vi "PD500 - PWM test cleanup_v2.vi"(0 "Control Board VISA":refnum<visa-resource-name>="ControlBoard", 1 "HMP VISA":refnum<visa-resource-name>, 2 "Board Selector":T1, 5 "error in (no error) 2":errorcluster) -> (12 "T6":dbl[](array[numeric]), 13 "T5":dbl[](array[numeric]), 15 "T4":dbl[](array[numeric]), 16 "T3":dbl[](array[numeric]), 17 "T2":dbl[](array[numeric]), 18 "T1":dbl[](array[numeric]), 19 "error out":errorcluster)   [LabVIEW 2022 SP3]
uses:
  Serial Board Com/Board Select.ctl
  HMP4000 Communication/HMP4040_ChannelControlAutomatic.ctl
  <vilib>/DAQmx/read.llb/DAQmx Read (Analog 1D Wfm NChan NSamp).vi
  <vilib>/DAQmx/miscellaneous.llb/DAQmx Fill In Error Info.vi
panel:
  out "subarray 12":dbl[](array[numeric])
  out "subarray 11":dbl[](array[numeric])
  out "subarray 10":dbl[](array[numeric])
  out "subarray 9":dbl[](array[numeric])
  out "subarray 8":dbl[](array[numeric])
  out "subarray 7":dbl[](array[numeric])
  out "subarray 6":dbl[](array[numeric])
  out "subarray 5":dbl[](array[numeric])
  out "subarray 4":dbl[](array[numeric])
  out "subarray 3":dbl[](array[numeric])
  out "subarray 2":dbl[](array[numeric])
  out "subarray":dbl[](array[numeric])
  out "Duty Cycle VISA Write":string[](array[string])
  out "Analysis Leg":i32
  out "Waveforms":T2
  out "Active Leg":i32
  # "Hugo: Needs Further Cleanup Regarding Data"
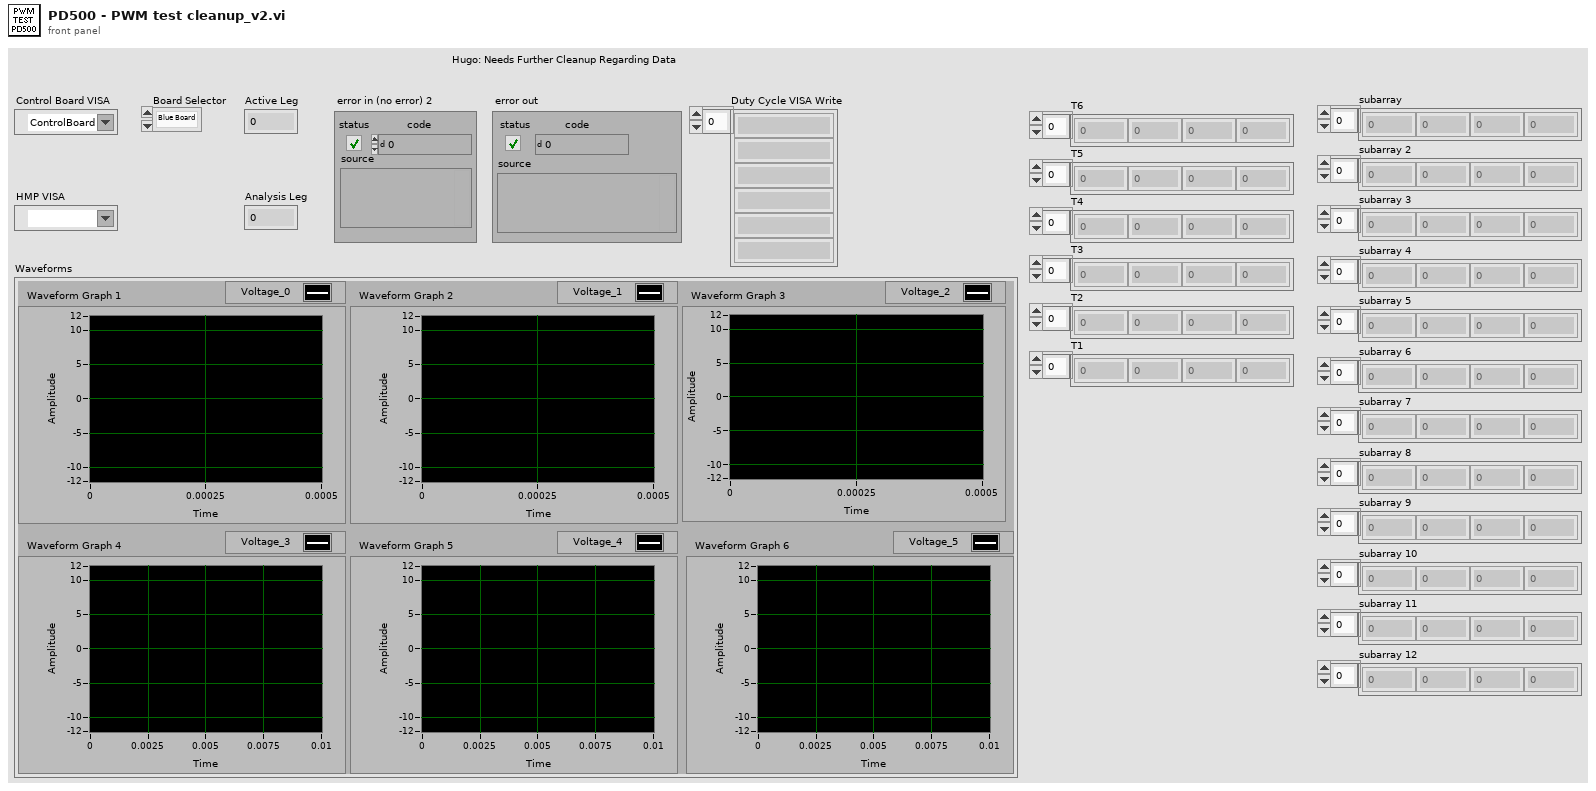
[diagram p1: front panel]
types:
  T1 = typedef "Board Select.ctl" = enum16{"Blue Board", "Green Board"}
  T2 = cluster{"Waveform Graph 1":waveform(dbl), "Waveform Graph 2":waveform(dbl), "Waveform Graph 3":waveform(dbl), "Waveform Graph 4":waveform(dbl), "Waveform Graph 5":waveform(dbl), "Waveform Graph 6":waveform(dbl)}
  T3 = typedef "HMP4040_ChannelControlAutomatic.ctl" = enum16{"Off", "Control Power", "HMP2020 Control + DC32V", "HMP2020 Control + DC8V", "HMP4040 Control + DC32V", "HMP4040 Control +DC8V", "HMP4040 Ch2 24V 4A"}
  T4 = cluster{"data[0]":waveform(dbl), "data[1]":waveform(dbl), "data[2]":waveform(dbl), "data[3]":waveform(dbl), "data[4]":waveform(dbl), "data[5]":waveform(dbl)}
  T5 = typedef "NI_Matrix.lvlib/RealMatrix.ctl" = dbl[][]
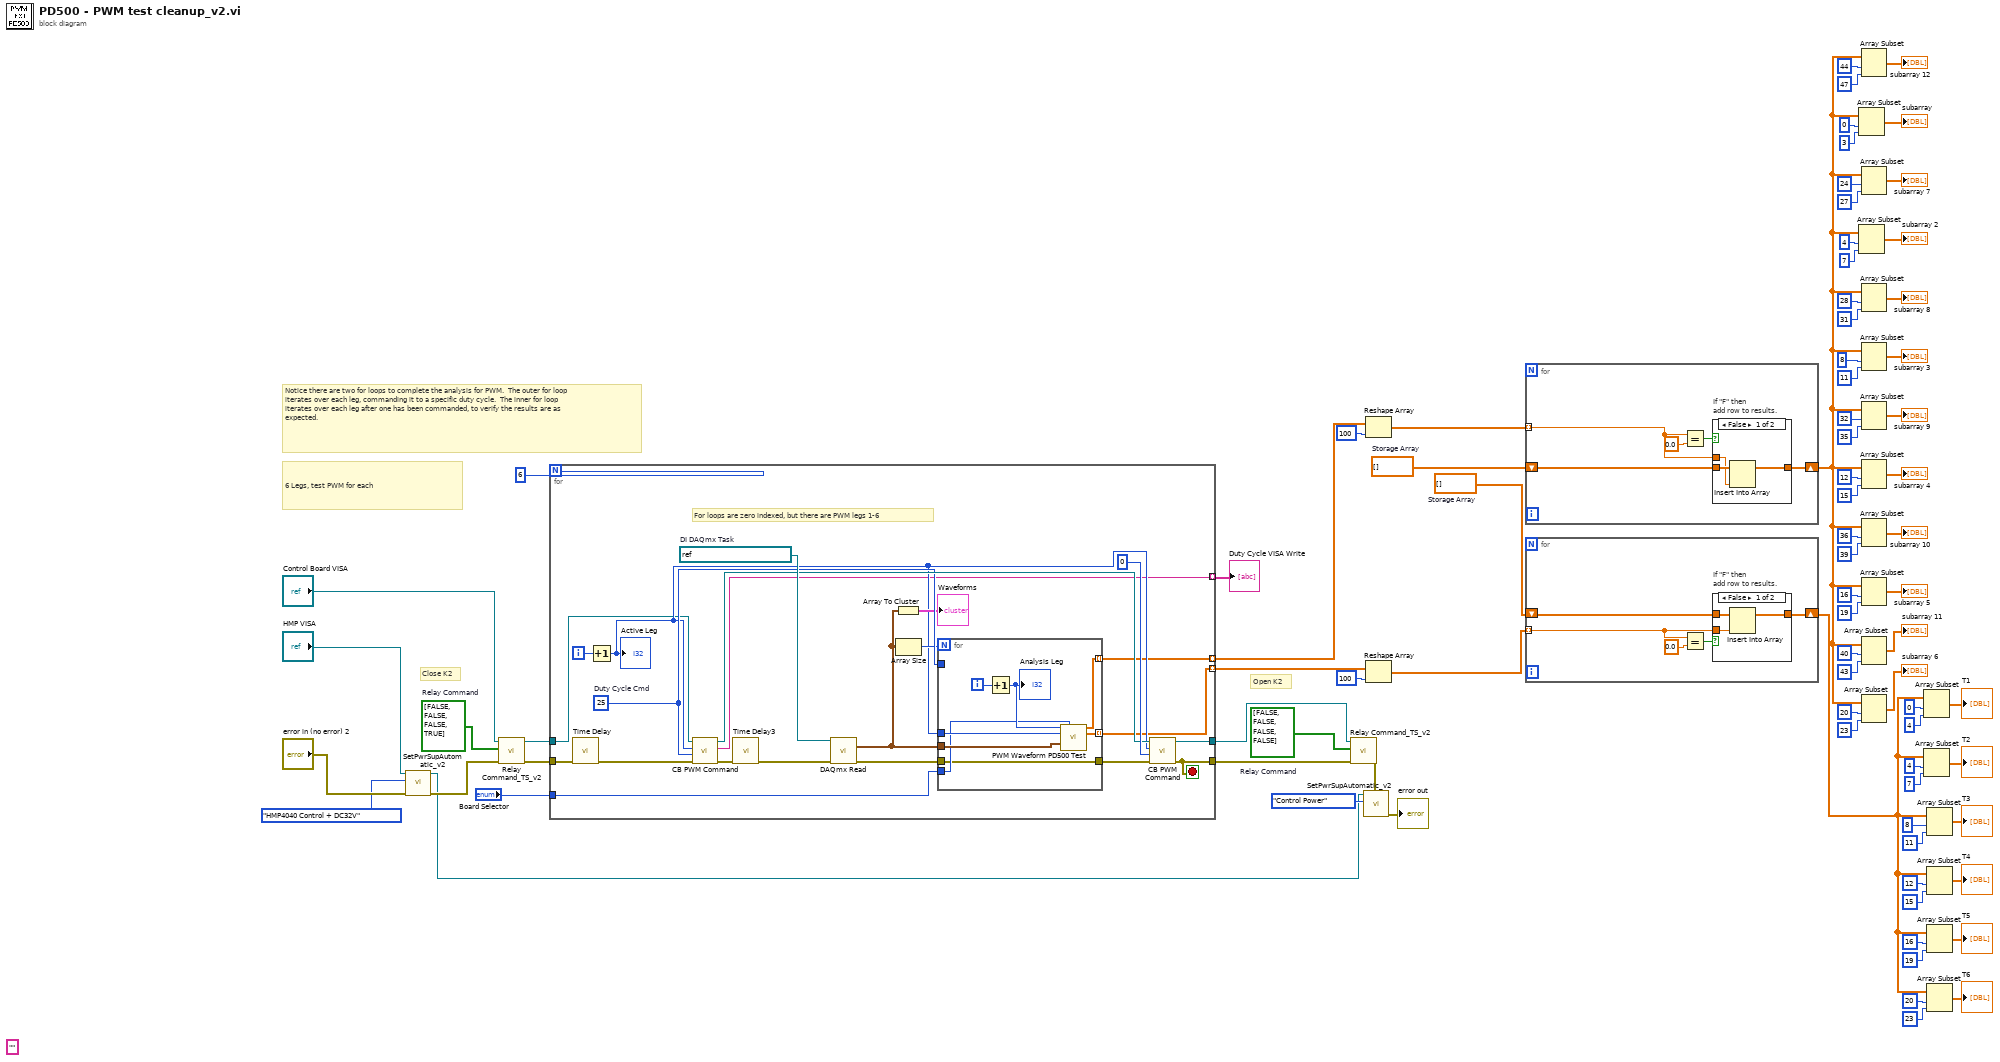
[diagram p0: block diagram]
diagram:
  w64 = dbl[] []  # Storage Array
  w66 = dbl[] []  # Storage Array
  w77 = bool[] [FALSE, FALSE, FALSE, TRUE]  # Relay Command
  w71 = bool[] [FALSE, FALSE, FALSE, FALSE]  # Relay Command
  (unwired) ""
  # "Close K2"
  # "Open K2"
  # "Notice there are two for loops to complete the analysis for PWM.  The outer for loop iterates over each leg, commanding it to a specific duty cycle.  The inner for loop iterates over each leg after one has been commanded, to verify the results are as expected."
  # "6 Legs, test PWM for each"
  n1 = call "SetPwrSupAutomatic_v2.vi"("error in (no error)"="error in (no error) 2", "Enum"=HMP4040_ChannelControlAutomatic."HMP4040 Control + DC32V", "HMP VISA"="HMP VISA") -> ("error out"=w75:errorcluster, "HMP VISA Out"=w4:refnum<visa-resource-name>)  [unwired: 7 in]
  n2 = call "Relay Command_TS_v2.vi"("error in (no error)"=w75, "Relay Command"=w77, "Control Board VISA"="Control Board VISA") -> ("error out"=w79:errorcluster, "VISA Refnum out"=w80:refnum<visa-resource-name>)  [unwired: 7 in]
  n3 = for {
    N: 6 -> [_]
    tunnel: [w99] -> w81
    tunnel: [w95] -> w3
    tunnel: w79 -> [w88]
    tunnel: w80 -> [w93]
    tunnel: [w90] -> w78 mode=indexing
    tunnel: "Board Selector" -> [w89]
    tunnel: [w86] -> w70 mode=indexing
    tunnel: [w85] -> w68 mode=indexing
    i -> [w100]
    stop <- w99 stop-if-true
    w101 = 25  # Duty Cycle Cmd
    w104 = refnum<k21> "FTS2_PWMInput_DG"  # DI DAQmx Task
    # "For loops are zero indexed, but there are PWM legs 1-6"
    n4 = call "Time Delay"("error in (no error)"=w88) -> ("error out"=w87:errorcluster)  [unwired: 10 in]
    n5 = Increment(x=w100) -> (x+1=w94:i32)
    "Active Leg" <- w94
    n6 = call "CB PWM Command.vi"("error in (no error)"=w87, "Duty Cycle"=w101, "Leg"=w94, "VISA Refnum in"=w93) -> ("error out"=w92:errorcluster, "read buffer"=w90:string, "VISA Refnum out"=w102:refnum<visa-resource-name>)  [unwired: 5 in]
    n7 = call "Time Delay3"("error in (no error)"=w92) -> ("error out"=w91:errorcluster)  [unwired: 10 in]
    n8 = call-poly <vilib>:"DAQmx Read.vi"("task/channels in"=w104, "error in"=w91) -> ("data"=w96:waveform(dbl)[], "error out"=w83:errorcluster)  [unwired: 11 in, 1 out]
    n9 = Array To Cluster(array=w96) -> (cluster=→"Waveforms":T4)
    n10 = Array Size(array=w96) -> (size(s)=w97:i32)
    n11 = for {
      N: w97 -> [_]
      tunnel: w101 -> [_]
      tunnel: w96 -> [w112]
      tunnel: w94 -> [w111]
      tunnel: w89 -> [w108]
      tunnel: [w107] -> w86 mode=indexing
      tunnel: [w106] -> w85 mode=indexing
      tunnel: [w105] -> w84
      tunnel: w83 -> [w105]
      i -> [w110]
      n12 = Increment(x=w110) -> (x+1=w109:i32)
      "Analysis Leg" <- w109
      n13 = call "PWM Waveform PD500 Test.vi"("Analysis Leg"=w109, "Board Selector"=w108, "Active Leg"=w111, "Waveform"=w112) -> ("Inactive Values"=w107:T5, "Active Values"=w106:T5)  [unwired: 10 in]
    }
    n14 = call "CB PWM Command.vi"("error in (no error)"=w84, "Duty Cycle"=0, "Leg"=w94, "VISA Refnum in"=w102) -> ("error out"=w99:errorcluster, "VISA Refnum out"=w95:refnum<visa-resource-name>)  [unwired: 5 in, 1 out]
  }
  "Duty Cycle VISA Write" <- w78
  n15 = call "Relay Command_TS_v2.vi"("error in (no error)"=w81, "Relay Command"=w71, "Control Board VISA"=w3) -> ("error out"=w74:errorcluster)  [unwired: 7 in, 1 out]
  n16 = call "SetPwrSupAutomatic_v2.vi"("error in (no error)"=w74, "Enum"=HMP4040_ChannelControlAutomatic."Control Power", "HMP VISA"=w4) -> ("error out"=→"error out":errorcluster)  [unwired: 7 in, 1 out]
  n17 = Reshape Array(w70, 100 ("dimension size")) -> (w65:dbl[])
  n18 = Reshape Array(w68, 100 ("dimension size")) -> (w63:dbl[])
  n19 = for {
    tunnel: w65 -> [w115] mode=indexing
    shift-right: [w116] -> w62
    shift-left: w66 -> [w117]
    n20 = Equal?(x=w115, y=0.0) -> (x = y?=w113:bool)
    n21 = case "If \"F\" then \nadd row to results." shown="False" w113 {
      tunnel: w117 -> [w120 w121]
      tunnel: w115 -> [w119 _]
      tunnel: [w118 w121] -> w116
      frame False {
        n22 = Insert Into Array(array=w120, new element=w119) -> (w118:dbl[])  [unwired: 1 in]
      }
      frame True {
      }
    }
  }
  n23 = for {
    tunnel: w63 -> [w124] mode=indexing
    shift-right: [w125] -> w13
    shift-left: w64 -> [w126]
    n24 = Equal?(x=w124, y=0.0) -> (x = y?=w122:bool)
    n25 = case "If \"F\" then \nadd row to results." shown="False" w122 {
      tunnel: w126 -> [w129 w130]
      tunnel: w124 -> [w128 _]
      tunnel: [w127 w130] -> w125
      frame False {
        n26 = Insert Into Array(array=w129, new element=w128) -> (w127:dbl[])  [unwired: 1 in]
      }
      frame True {
      }
    }
  }
  n27 = Array Subset(array=w62, index=0, length=3) -> (→"subarray":dbl[])
  n28 = Array Subset(array=w62, index=4, length=7) -> (→"subarray 2":dbl[])
  n29 = Array Subset(array=w62, index=44, length=47) -> (→"subarray 12":dbl[])
  n30 = Array Subset(array=w62, index=24, length=27) -> (→"subarray 7":dbl[])
  n31 = Array Subset(array=w62, index=28, length=31) -> (→"subarray 8":dbl[])
  n32 = Array Subset(array=w62, index=8, length=11) -> (→"subarray 3":dbl[])
  n33 = Array Subset(array=w62, index=32, length=35) -> (→"subarray 9":dbl[])
  n34 = Array Subset(array=w62, index=12, length=15) -> (→"subarray 4":dbl[])
  n35 = Array Subset(array=w62, index=36, length=39) -> (→"subarray 10":dbl[])
  n36 = Array Subset(array=w62, index=16, length=19) -> (→"subarray 5":dbl[])
  n37 = Array Subset(array=w62, index=40, length=43) -> (→"subarray 11":dbl[])
  n38 = Array Subset(array=w62, index=20, length=23) -> (→"subarray 6":dbl[])
  n39 = Array Subset(array=w13, index=0, length=4) -> (→"T1":dbl[])
  n40 = Array Subset(array=w13, index=4, length=7) -> (→"T2":dbl[])
  n41 = Array Subset(array=w13, index=8, length=11) -> (→"T3":dbl[])
  n42 = Array Subset(array=w13, index=12, length=15) -> (→"T4":dbl[])
  n43 = Array Subset(array=w13, index=16, length=19) -> (→"T5":dbl[])
  n44 = Array Subset(array=w13, index=20, length=23) -> (→"T6":dbl[])
